vi "ATTN.vi"(8 "error in (no error)":errorcluster, 10 "Attn":u32(ring) items=["Off", "On"], 11 "VISA resource name":refnum<visa-resource-name>) -> (0 "error out":errorcluster, 3 "VISA resource name out":refnum<visa-resource-name>)   [LabVIEW 2009, in "Newport 1830-C.lvlib"]
doc: "Attenuator\n0=OFF\n1=ON"
uses:
  Newport 1830-C.lvlib
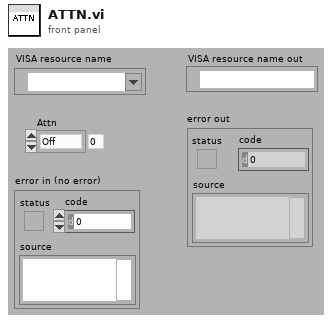
[diagram p1: front panel]
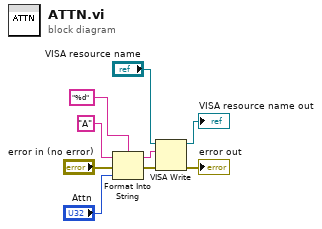
[diagram p0: block diagram]
diagram:
  n1 = Format Into String(format string="%d", initial string="A" ("command"), error in="error in (no error)", "Attn") -> (resulting string=w5:string, error out=w6:errorcluster)
  n2 = VISA Write(VISA resource name="VISA resource name", write buffer=w5, error in (no error)=w6) -> (VISA resource name out=→"VISA resource name out":refnum<visa-resource-name>, error out=→"error out":errorcluster)  [unwired: 1 out]
